vi "Decode Statusword.vi"(1 "Data":u16 format="%b") -> (0 "Status":T1)   [LabVIEW 2016]
uses:
  Statusword.ctl
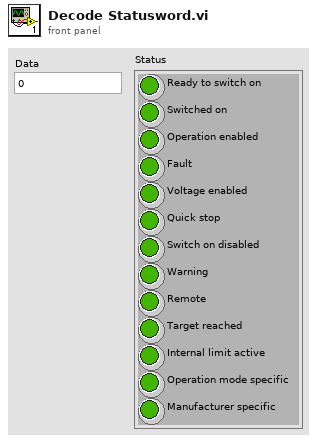
[diagram p1: front panel]
types:
  T1 = typedef "Statusword.ctl" = cluster{"Ready to switch on":bool, "Switched on":bool, "Operation enabled":bool, "Fault":bool, "Voltage enabled":bool, "Quick stop":bool, "Switch on disabled":bool, "Warning":bool, "Remote":bool, "Target reached":bool, "Internal limit active":bool, "Operation mode specific":bool, "Manufacturer specific":bool}
  T2 = cluster{"Boolean array[0]":bool, "Boolean array[1]":bool, "Boolean array[2]":bool, "Boolean array[3]":bool, "Boolean array[4]":bool, "Boolean array[5]":bool, "Boolean array[6]":bool, "Boolean array[7]":bool, "Boolean array[8]":bool, "Boolean array[9]":bool, "Boolean array[10]":bool, "Boolean array[11]":bool, "Boolean array[12]":bool, "Boolean array[13]":bool, "Boolean array[14]":bool, "Boolean array[15]":bool}
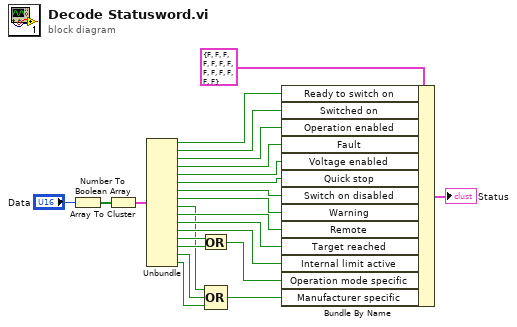
[diagram p0: block diagram]
diagram:
  n1 = Number To Boolean Array(number="Data") -> (Boolean array=w23:bool[])
  n2 = Array To Cluster(array=w23) -> (cluster=w22:T2)
  n3 = Unbundle(w22) -> ("Boolean array[0]"=w18:bool, "Boolean array[1]"=w17:bool, "Boolean array[2]"=w16:bool, "Boolean array[3]"=w15:bool, "Boolean array[4]"=w14:bool, "Boolean array[5]"=w13:bool, "Boolean array[6]"=w12:bool, "Boolean array[7]"=w11:bool, "Boolean array[8]"=w5:bool, "Boolean array[9]"=w10:bool, "Boolean array[10]"=w9:bool, "Boolean array[11]"=w8:bool, "Boolean array[12]"=w7:bool, "Boolean array[13]"=w6:bool, "Boolean array[14]"=w4:bool, "Boolean array[15]"=w3:bool)
  n4 = Or(x=w7, y=w6) -> (x .or. y?=w1:bool)
  n5 = Compound Arithmetic op=OR(w5, w4, w3) -> (w2:bool)
  n6 = Bundle By Name(cluster=T1 {"Ready to switch on"=FALSE, "Switched on"=FALSE, "Operation enabled"=FALSE, "Fault"=FALSE, "Voltage enabled"=FALSE, "Quick stop"=FALSE, "Switch on disabled"=FALSE, "Warning"=FALSE, "Remote"=FALSE, "Target reached"=FALSE, "Internal limit active"=FALSE, "Operation mode specific"=FALSE, "Manufacturer specific"=FALSE} ("Status"), "Ready to switch on"=w18, "Switched on"=w17, "Operation enabled"=w16, "Fault"=w15, "Voltage enabled"=w14, "Quick stop"=w13, "Switch on disabled"=w12, "Warning"=w11, "Remote"=w10, "Target reached"=w9, "Internal limit active"=w8, "Operation mode specific"=w1, "Manufacturer specific"=w2) -> (→"Status":T1)
